vi "Write Detector Config.vi"(8 "error in (no error)":errorcluster, 10 "Detector Config":T1={"Detector"=0, "Offsets"=[[0, 0, 0, 0, 0, 0, 0, 0, 0, 0, 0, 0, 0, 0, 0, 0, 0, 0, 0, 0, 0, 0, 0, 0, 0, 0, 0, 0, 0, 0, 0, 0]], "Detector Computer"={"Machine"="192.168.121.11", "Password"="rSL!nux23456", "FITS File Path"="", "Port"=44444, "Header Path"="", "Name"=""}, "FITS hdr template0"=path "", "FITS hdr template1"=path "", "FITS Data File Path"=path "", "FITS Detector Settings"={"Exp Time Short"=0.0, "# of Frames"=0.0, "Exp Time Long"=0.0, "# of Groups"=0.0, "Object Name"="", "Object"="", "Obs Type"="", "Image Type"="", "Observer"="", "Observer Affiliation"=""}, "Sim Folder"=path "", "Integration Mode"=enum."Ramp", "Integration Time"=0.0, "Frame Int Time"=0.0} {"Offsets" format="%04x"; "Detector" items=["0", "1", "2"]}, 11 "Detector Simulator in":refnum<class "Detector Simulator.lvclass">) -> (0 "error out":errorcluster, 3 "Detector Simulator out":refnum<class "Detector Simulator.lvclass">)   [LabVIEW 2024, in "Detector Simulator.lvclass"]
uses:
  Detector Simulator.lvclass
  RIMAS Detector Config.ctl
  RIMAS Detector Server Config.ctl
  RIMAS Observation Config.ctl
  Detector Class/Detector enum Detector Integration Mode.ctl
  Detector Simulator.lvclass/Detector Simulator.ctl
  Detector Class/Detector Class.lvclass
panel:
  # "sec"
  # "sec"
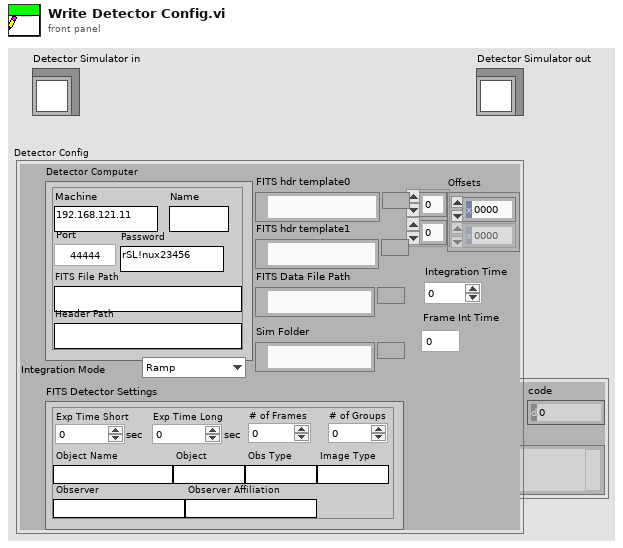
[diagram p1: front panel]
types:
  T1 = typedef "RIMAS Detector Config.ctl" = cluster{"Detector":u16, "Offsets":u16[][], "Detector Computer":T2, "FITS hdr template0":path, "FITS hdr template1":path, "FITS Data File Path":path, "FITS Detector Settings":T3, "Sim Folder":path, "Integration Mode":T4, "Integration Time":dbl, "Frame Int Time":dbl}
  T2 = typedef "RIMAS Detector Server Config.ctl" = cluster{"Machine":string, "Password":string, "FITS File Path":string, "Port":u16, "Header Path":string, "Name":string}
  T3 = typedef "RIMAS Observation Config.ctl" = cluster{"Exp Time Short":dbl, "# of Frames":dbl, "Exp Time Long":dbl, "# of Groups":dbl, "Object Name":string, "Object":string, "Obs Type":string, "Image Type":string, "Observer":string, "Observer Affiliation":string}
  T4 = typedef "Detector enum Detector Integration Mode.ctl" = enum16{"Ramp", "CDS", "FOWLER2", "FOWLER4", "FOWLER8", "FOWLER16", "Raw"}
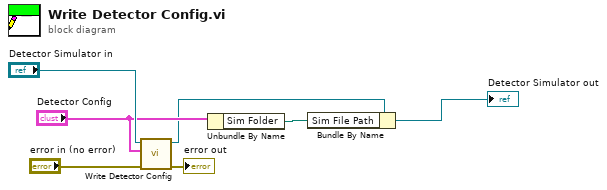
[diagram p0: block diagram]
diagram:
  n1 = call-parent "Write Detector Config.vi"("error in (no error)"="error in (no error)", "Detector Config"="Detector Config", "Detector Class in"="Detector Simulator in") -> ("error out"=→"error out":errorcluster, "Detector Class out"=w2:refnum<class "Detector Simulator.lvclass">)  [unwired: 7 in]
  n2 = Unbundle By Name("Detector Config") -> ("Sim Folder"=w3:path)
  n3 = Bundle By Name(cluster=w2, "Sim File Path"=w3) -> (→"Detector Simulator out":refnum<class "Detector Simulator.lvclass">)
